vi "RT Host - calc perp x & y.vi"(7 "Perp Dist Global W/S (mm)":dbl, 8 "error in (no error)":errorcluster, 10 "Previous Target Global W/S Pos (mm)":dbl[](array[numeric])=[0.0, -90.0], 11 "Target Global W/S Pos (mm)":dbl[](array[numeric])=[0.0, -90.0]) -> (0 "error out":errorcluster, 1 "Gradient":dbl, 2 "Perp Y Adjustment (mm)":dbl, 3 "Perp X Adjustment (mm)":dbl)   [LabVIEW 2017]
doc: "This subVI calculates the perpendicular difference between the allowable dead zone and current perpendicular distance from the desired trajectory."
panel:
  # "Inputs"
  # "Outputs"
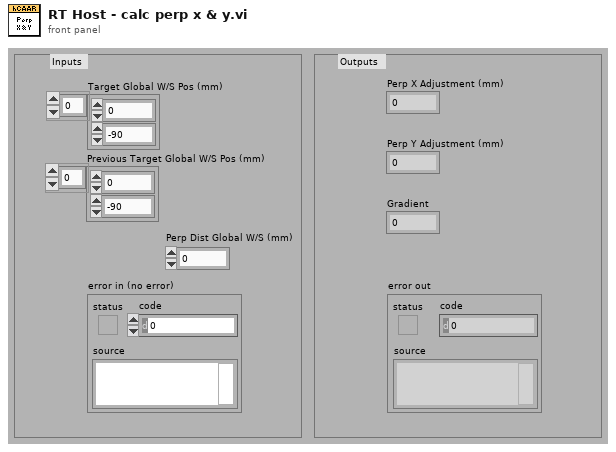
[diagram p1: front panel]
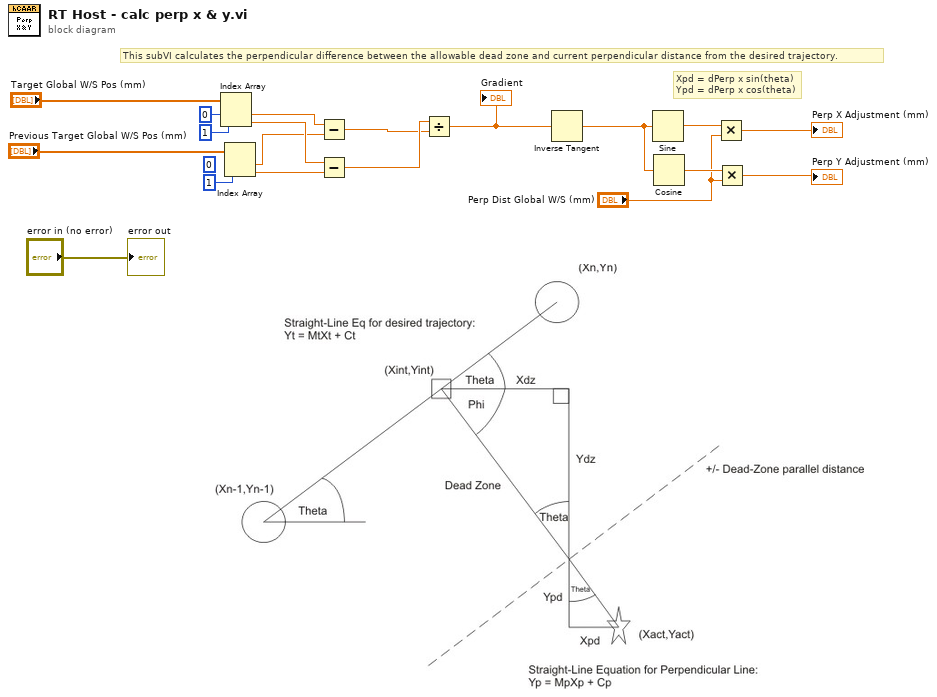
[diagram p0: block diagram]
diagram:
  (unwired) 0 ("index")
  # "Xpd = dPerp x sin(theta)\nYpd = dPerp x cos(theta)"
  # "This subVI calculates the perpendicular difference between the allowable dead zone and current perpendicular distance from the desired trajectory."
  n1 = Index Array(array="Target Global W/S Pos (mm)", index #1=0 ("index"), index #2=1 ("index")) -> (element #1=w12:dbl, element #2=w15:dbl)
  n2 = Index Array(array="Previous Target Global W/S Pos (mm)", index #2=1 ("index")) -> (element #1=w13:dbl, element #2=w14:dbl)  [unwired: 1 in]
  n3 = Subtract(x=w12, y=w13) -> (x-y=w16:dbl)
  n4 = Subtract(x=w15, y=w14) -> (x-y=w17:dbl)
  n5 = Divide(x=w17, y=w16) -> (x/y=w6:dbl)
  "Gradient" <- w6
  n6 = Inverse Tangent(1:w6) -> (0:w5:dbl)
  n7 = Sine(x=w5) -> (sin(x)=w18:dbl)
  n8 = Cosine(x=w5) -> (cos(x)=w19:dbl)
  n9 = Multiply(x=w18, y="Perp Dist Global W/S (mm)") -> (x*y=→"Perp X Adjustment (mm)":dbl)
  n10 = Multiply(x=w19, y="Perp Dist Global W/S (mm)") -> (x*y=→"Perp Y Adjustment (mm)":dbl)
  "error out" <- "error in (no error)"
